vi "Draw Circle.vi"(1 "radius":dbl, 2 "Pos XY":dbl[][](array[numeric])) -> (0 "Bound out":T1)   [LabVIEW 2016]
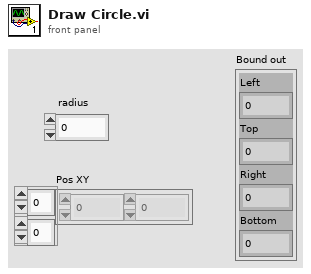
[diagram p1: front panel]
types:
  T1 = cluster{"Left":i32, "Top":i32, "Right":i32, "Bottom":i32}
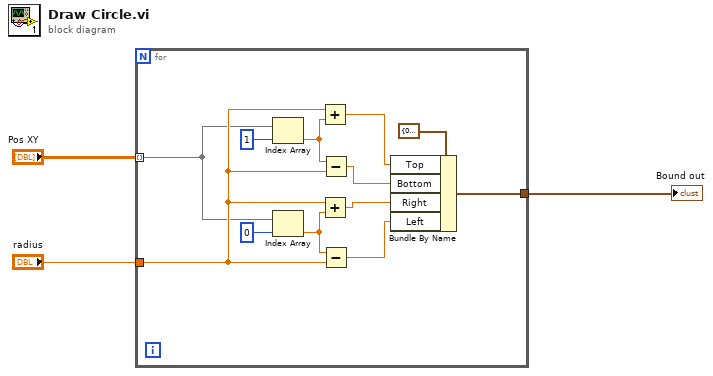
[diagram p0: block diagram]
diagram:
  n1 = for {
    tunnel: "radius" -> [w15]
    tunnel: "Pos XY" -> [w14] mode=indexing
    tunnel: [w4] -> w1
    n2 = Index Array(array=w14, index=1 ("索引")) -> (element=w12:dbl)
    n3 = Index Array(array=w14, index=0 ("索引")) -> (element=w11:dbl)
    n4 = Add(x=w15, y=w12) -> (x+y=w8:dbl)
    n5 = Add(x=w15, y=w11) -> (x+y=w6:dbl)
    n6 = Subtract(x=w12, y=w15) -> (x-y=w7:dbl)
    n7 = Subtract(x=w11, y=w15) -> (x-y=w5:dbl)
    n8 = Bundle By Name(cluster=T1 {"Left"=0, "Top"=0, "Right"=0, "Bottom"=0} ("Bounding Rectangle"), "Top"=w8, "Bottom"=w7, "Right"=w6, "Left"=w5) -> (w4:T1)
  }
  "Bound out" <- w1
